vi "sv_Get Samples to Next Zero Crossing .vi"(4 "write index - block size":u32, 6 "phase":dbl format="%.2f", 7 "frequency to generate [Hz]":dbl format="%.2f", 10 "AI sampling frequency":dbl format="%.2f", 11 "indice computations in":T1) -> (2 "dup AI sampling frequency":dbl format="%.2f", 3 "indice computations in":T1)   [LabVIEW 2017, in "SoundVib_SweptSine.lvlib"]
uses:
  <vilib>/addons/Sound and Vibration/svt_Swept Sine/SoundVib_SweptSine.lvlib
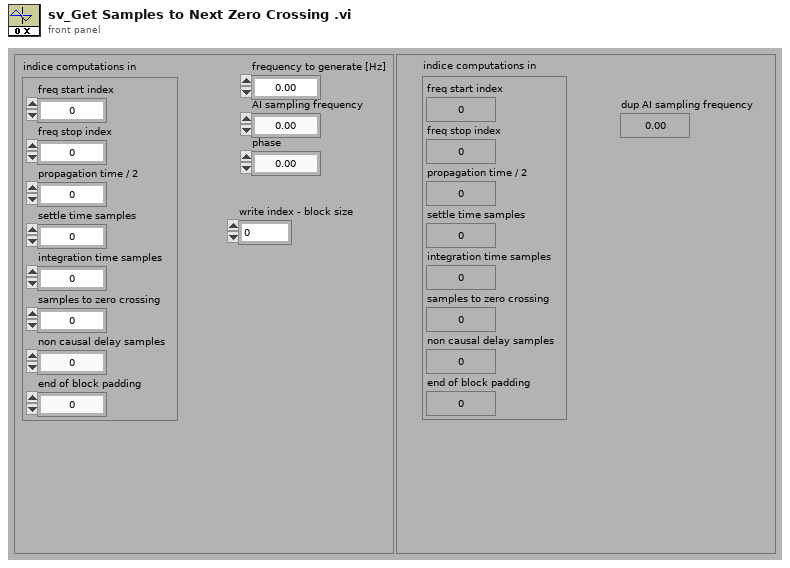
[diagram p1: front panel]
types:
  T1 = cluster{"freq start index":u32, "freq stop index":u32, "propagation time / 2":u32, "settle time samples":u32, "integration time samples":u32, "samples to zero crossing":u32, "non causal delay samples":u32, "end of block padding":u32}
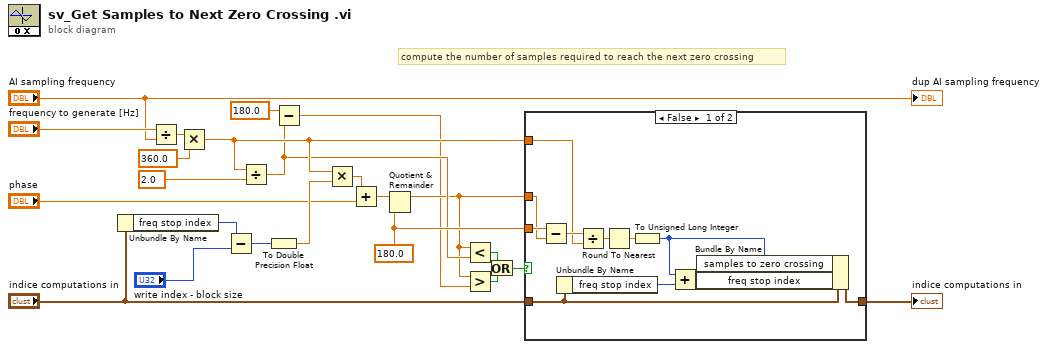
[diagram p0: block diagram]
diagram:
  w20 = 180.0 ("y")
  # "compute the number of samples required to reach the next zero crossing"
  n1 = Unbundle By Name("indice computations in") -> ("freq stop index"=w3:u32)
  n2 = Divide(x="frequency to generate [Hz]", y="AI sampling frequency") -> (x/y=w22:dbl)
  n3 = Multiply(x=w22, y=360.0 ("x")) -> (x*y=w12:dbl)
  n4 = Subtract(x=w3, y="write index - block size") -> (x-y=w1:u32)
  n5 = Divide(x=w12, y=2.0) -> (x/y=w9:dbl)
  n6 = To Double Precision Float(number=w1) -> (double precision float=w18:dbl)
  n7 = Subtract(x=180.0 ("y"), y=w9) -> (x-y=w7:dbl)
  n8 = Multiply(x=w12, y=w18) -> (x*y=w21:dbl)
  n9 = Add(x=w21, y="phase") -> (x+y=w15:dbl)
  n10 = Quotient & Remainder(x=w15, y=w20) -> (x-y*floor(x/y)=w8:dbl)  [unwired: 1 out]
  n11 = Less?(x=w8, y=w9) -> (x < y?=w6:bool)
  n12 = Greater?(x=w8, y=w7) -> (0:w5:bool)
  n13 = Or(x=w6, y=w5) -> (x .or. y?=w4:bool)
  n14 = case shown="False" w4 {
    tunnel: w20 -> [w34 _]
    tunnel: w12 -> [w32 _]
    tunnel: w8 -> [w30 _]
    tunnel: "indice computations in" -> [w26 w35]
    tunnel: [w25 w35] -> w13
    frame False {
      n15 = Subtract(x=w34, y=w30) -> (x-y=w33:dbl)
      n16 = Unbundle By Name(w26) -> ("freq stop index"=w27:u32)
      n17 = Divide(x=w33, y=w32) -> (x/y=w31:dbl)
      n18 = Round To Nearest(number=w31) -> (nearest integer value=w29:dbl)
      n19 = To Unsigned Long Integer(number=w29) -> (unsigned 32bit integer=w24:u32)
      n20 = Add(x=w24, y=w27) -> (x+y=w28:u32)
      n21 = Bundle By Name(cluster=w26, "samples to zero crossing"=w24, "freq stop index"=w28) -> (w25:T1)
    }
    frame True {
    }
  }
  "indice computations in" <- w13
  "dup AI sampling frequency" <- "AI sampling frequency"
